vi "VAT_valve_read_write.vi"(0 "VAT Valve COM port":refnum<visa-resource-name>, 2 "Write String":string, 11 "error in (no error)":errorcluster) -> (4 "VAT Valve COM port out":refnum<visa-resource-name>, 13 "Read String":string, 15 "error out":errorcluster)   [LabVIEW 2019]
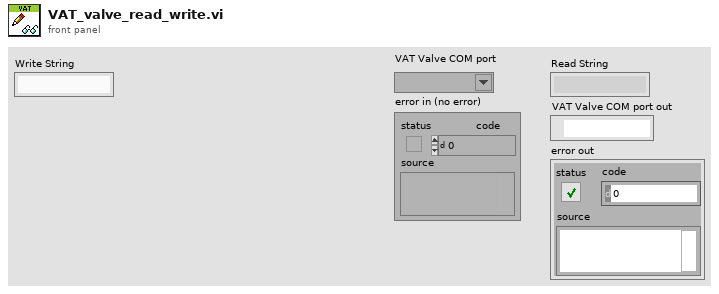
[diagram p1: front panel]
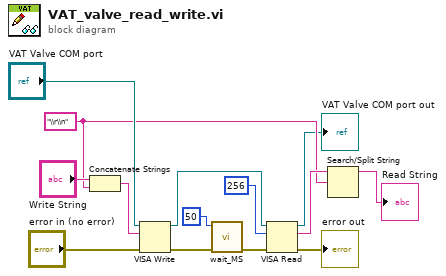
[diagram p0: block diagram]
diagram:
  w4 = "\\r\\n" ("string")
  n1 = Concatenate Strings("Write String", w4) -> (w11:string)
  n2 = VISA Write(VISA resource name="VAT Valve COM port", write buffer=w11, error in (no error)="error in (no error)") -> (VISA resource name out=w6:refnum<visa-resource-name>, error out=w10:errorcluster)  [unwired: 1 out]
  n3 = call "wait_MS.vi"("error in (no error)"=w10, "milliseconds to wait"=u32 50) -> ("error out"=w9:errorcluster)  [unwired: 9 in]
  n4 = VISA Read(VISA resource name=w6, byte count=u32 256, error in (no error)=w9) -> (VISA resource name out=→"VAT Valve COM port out":refnum<visa-resource-name>, read buffer=w5:string, error out=→"error out":errorcluster)  [unwired: 1 out]
  n5 = Search/Split String(string=w5, search string/char (-)=w4) -> (substring before match=→"Read String":string)  [unwired: 1 in, 2 out]
